vi "test Add RAF Channel.vi"(8 "error in (no error)":errorcluster, 11 "TestCase in":refnum<class "Switch Scripting Test Case.lvclass">) -> (0 "error out":errorcluster, 3 "TestCase out":refnum<class "Switch Scripting Test Case.lvclass">)   [LabVIEW 2017, in "Switch Scripting Test Case.lvclass"]
uses:
  Switch Scripting Test Case.lvclass
  Scripting/Channel States.ctl
  Scripting/Routing State.ctl
  Scripting/Routing Channel/Connection.ctl
  Shared/Routing and Faulting Custom Device Settings.ctl
  Switch Scripting Test Case.lvclass/Switch Scripting Test Case.ctl
  <vilib>/addons/_JKI Toolkits/VI Tester/TestCase.llb/TestCase.lvclass
  Scripting/Switch Scripting.lvlib
  Shared/Switch Shared.lvlib
  C:/Program Files (x86)/National Instruments/LabVIEW 2017/vi.lib/addons/_JKI Toolkits/VI Tester/TestCase.llb/TestCase.lvclass
panel:
  in  "Save?":bool
  out "Output Filename":string
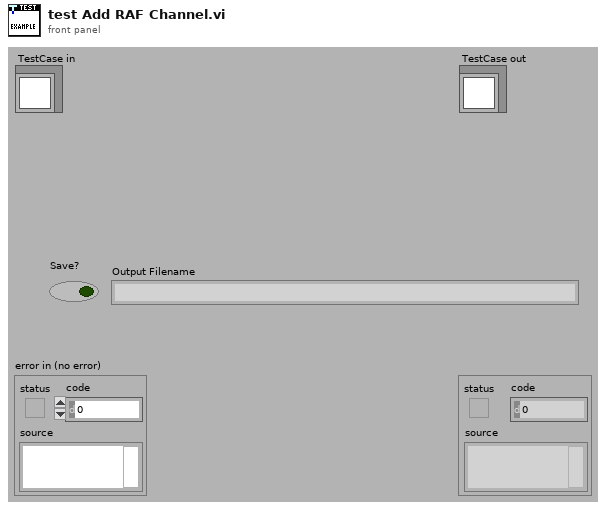
[diagram p1: front panel]
types:
  T1 = typedef "Switch Scripting.lvlib/Connection.ctl" = cluster{"Source":string, "Destination":string}
  T2 = typedef "Switch Shared.lvlib/Routing and Faulting Custom Device Settings.ctl" = cluster{"Name":string}
  T3 = typedef "Switch Scripting.lvlib/Channel States.ctl" = T4[]
  T4 = typedef "Switch Scripting.lvlib/Routing State.ctl" = cluster{"name":string, "value":i32, "Connection List":T1[]}
  T5 = typedef "Custom Device API.lvlib/Custom Device Item Ref.ctl" = u64
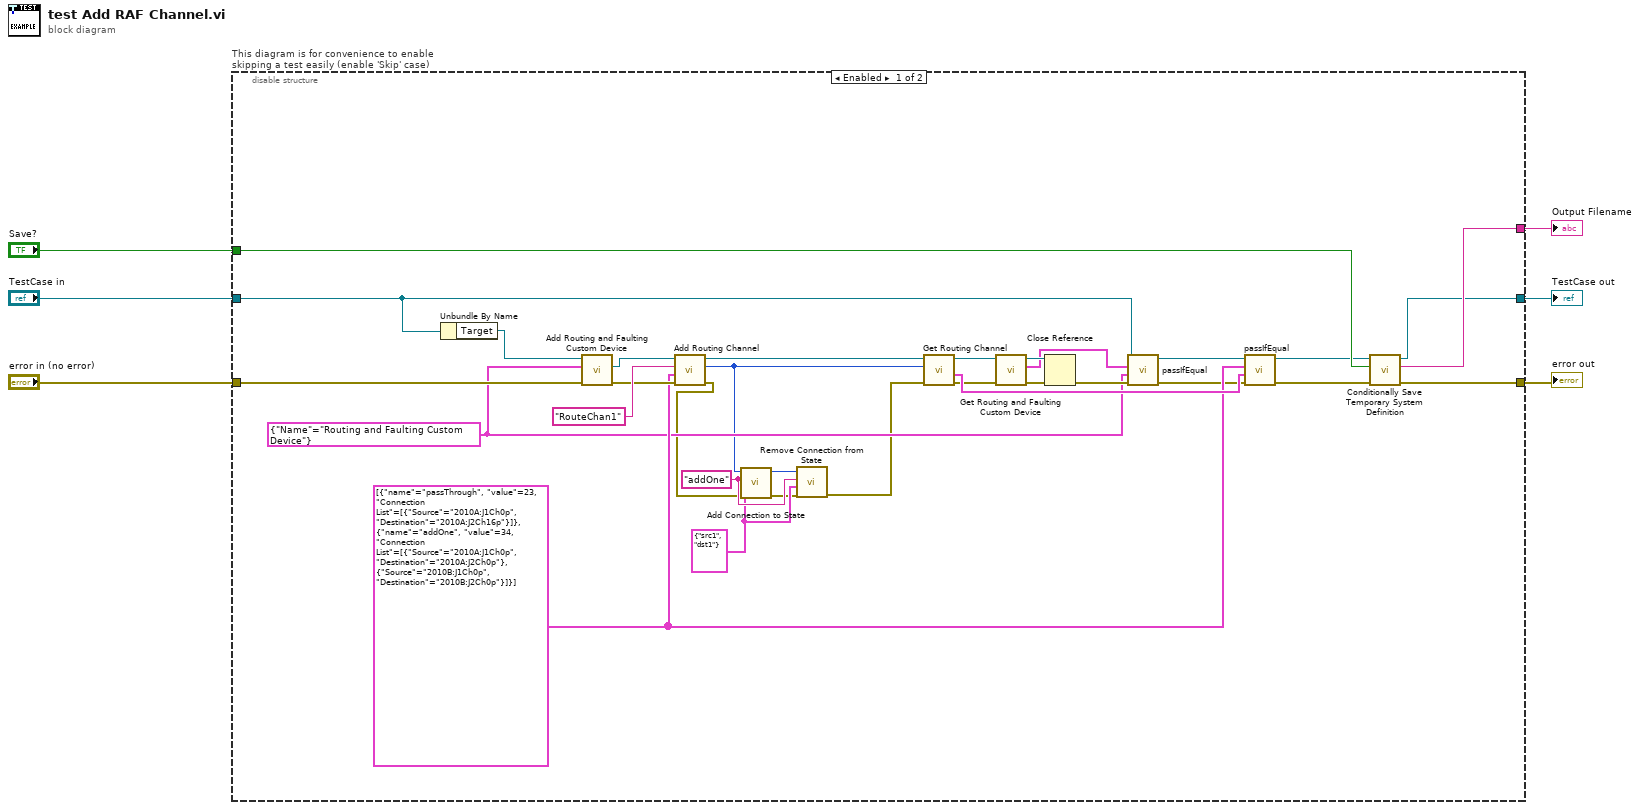
[diagram p0: block diagram]
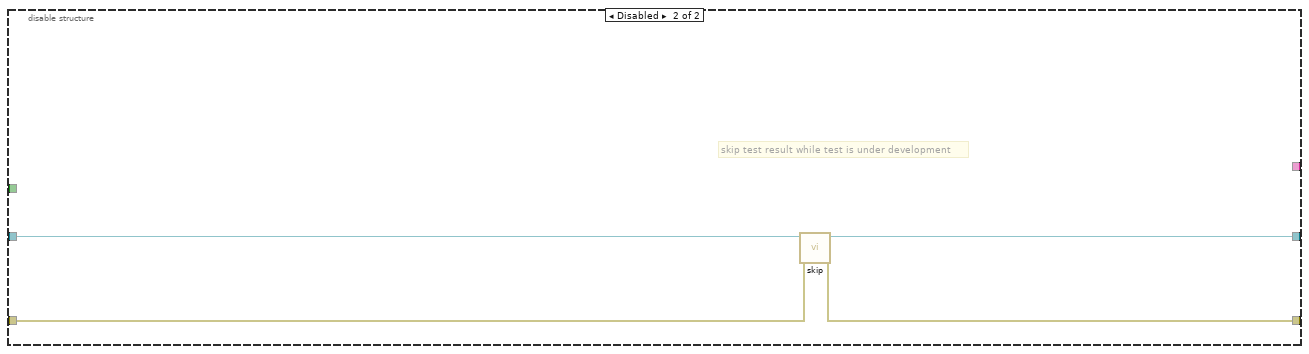
[diagram p2: hidden frame]
diagram:
  n1 = disable-structure "This diagram is for convenience to enable skipping a test easily (enable 'Skip' case)" shown="Enabled" {
    disable-tunnel: "TestCase in" -> [w31 w41]
    disable-tunnel: [w29 w39] -> w3
    disable-tunnel: [w36 w40] -> w5
    disable-tunnel: "error in (no error)" -> [w37 w38]
    disable-tunnel: [w35 _] -> w2
    disable-tunnel: "Save?" -> [w34 _]
    frame Enabled {
      w10 = T1 {"Source"="src1", "Destination"="dst1"} ("connection")
      w11 = "addOne" ("state name")
      w16 = T2 {"Name"="Routing and Faulting Custom Device"} ("Routing and Faulting Custom Device Settings")
      w17 = T3 [{"name"="passThrough", "value"=23, "Connection List"=[{"Source"="2010A:J1Ch0p", "Destination"="2010A:J2Ch16p"}]}, {"name"="addOne", "value"=34, "Connection List"=[{"Source"="2010A:J1Ch0p", "Destination"="2010A:J2Ch0p"}, {"Source"="2010B:J1Ch0p", "Destination"="2010B:J2Ch0p"}]}] ("Channel States")
      n2 = Unbundle By Name(w31) -> ("Target"=w30:refnum<k24>)
      n3 = call "Add Routing and Faulting Custom Device.vi"("error in (no error)"=w37, "Settings"=w16, "Target in"=w30) -> ("error out"=w24:errorcluster, "RAF Custom Device"=w25:refnum<k24>)  [unwired: 6 in, 1 out]
      n4 = call "Add Routing Channel.vi"("error in (no error)"=w24, "Channel States"=w17, "Channel Name"="RouteChan1", "RAF Custom Device in"=w25) -> ("error out"=w7:errorcluster, "Channel Ref"=w15:T5, "RAF Custom Device out"=w21:refnum<k24>)  [unwired: 5 in]
      n5 = call "Add Connection to State.vi"("error in (no error)"=w7, "Connection"=w10, "State"=w11, "Channel Ref in"=w15) -> ("error out"=w8:errorcluster, "Channel Ref out"=w12:T5)  [unwired: 6 in]
      n6 = call "Remove Connection from State.vi"("error in (no error)"=w8, "Connection"=w10, "State"=w11, "Channel Ref in"=w12) -> ("error out"=w9:errorcluster)  [unwired: 5 in, 2 out]
      n7 = call "Get Routing Channel.vi"("error in (no error)"=w9, "Channel Ref"=w15, "RAF Custom Device in"=w21) -> ("error out"=w19:errorcluster, "Channel States"=w22:T3, "RAF Custom Device out"=w20:refnum<k24>)  [unwired: 5 in, 1 out]
      n8 = call "Get Routing and Faulting Custom Device.vi"("error in (no error)"=w19, "RAF Custom Device in"=w20) -> ("error out"=w28:errorcluster, "Settings"=w32:T2, "RAF Custom Device out"=w33:refnum<k24>)  [unwired: 7 in]
      n9 = Close Reference(reference=w33, error in (no error)=w28) -> (error out=w27:errorcluster)
      n10 = call-dynamic "passIfEqual.vi"("error in (no error)"=w27, "y"=w16, "x"=w32, "TestCase in"=w31) -> ("error out"=w13:errorcluster, "TestCase out"=w14:refnum<class "Switch Scripting Test Case.lvclass">)  [unwired: 6 in]
      n11 = call-dynamic "passIfEqual.vi"("error in (no error)"=w13, "y"=w22, "x"=w17, "TestCase in"=w14) -> ("error out"=w23:errorcluster, "TestCase out"=w18:refnum<class "Switch Scripting Test Case.lvclass">)  [unwired: 6 in]
      n12 = call "Conditionally Save Temporary System Definition.vi"("error in (no error)"=w23, "Save?"=w34, "Test Case"=w18) -> ("error out"=w36:errorcluster, "filename"=w35:string, "Test Case"=w29:refnum<class "Switch Scripting Test Case.lvclass">)  [unwired: 6 in]
    }
    frame Disabled {
      # "skip test result while test is under development"
      n13 = call <vilib>:"skip.vi"("error in (no error)"=w38, "TestCase in"=w41) -> ("error out"=w40:errorcluster, "TestCase out"=w39:refnum<class "Switch Scripting Test Case.lvclass">)  [unwired: 8 in]
    }
  }
  "error out" <- w5
  "TestCase out" <- w3
  "Output Filename" <- w2
